vi "Info from Source.vi"(8 "error in (no error)":errorcluster, 9 "Branch (Default)":string, 10 "Source":string, 11 "Package in":refnum<class "Package.lvclass">) -> (0 "error out":errorcluster, 2 "Package Info":T1, 3 "Package out":refnum<class "Package.lvclass">)   [LabVIEW 2020, in "GPack.lvlib" / "Package.lvclass"]
uses:
  Package.lvclass
  Package Info.ctl
  GPack.lvlib
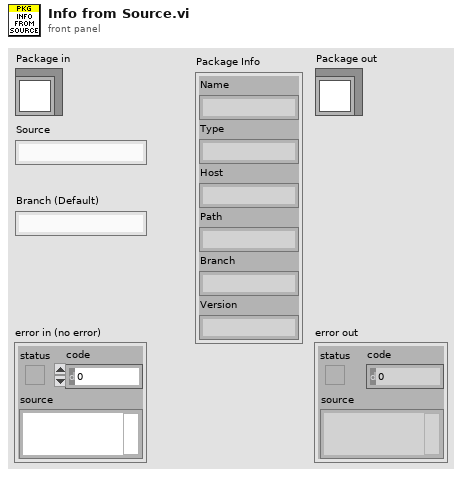
[diagram p1: front panel]
types:
  T1 = typedef "GPack.lvlib/Package Info.ctl" = cluster{"Name":string, "Type":string, "Host":string, "Path":string, "Branch":string, "Version":string}
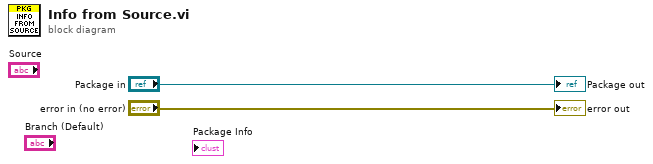
[diagram p0: block diagram]
diagram:
  "error out" <- "error in (no error)"
  "Package out" <- "Package in"
